vi "VirtualTestInstrument.vi"(8 "error in (no error)":errorcluster, 10 "Message":T1, 11 "RemoteControl":refnum<class "RemoteControl.lvclass">) -> (0 "error out":errorcluster, 2 "processed Message":T1, 3 "RemoteControl":refnum<class "RemoteControl.lvclass">)   [LabVIEW 2016, in "RemoteControl.lvclass"]
uses:
  RemoteControl.lvclass
  Typedefs/Message--Cluster.ctl
  RemoteControl.lvclass/RemoteControl.ctl
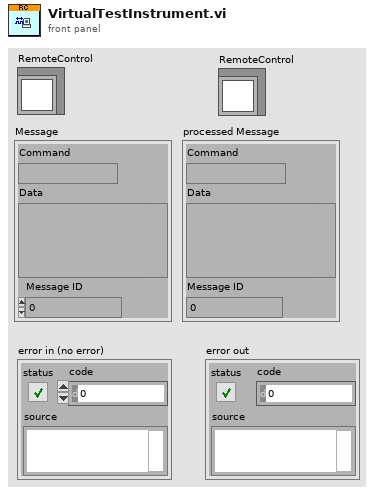
[diagram p1: front panel]
types:
  T1 = typedef "RemoteControl.lvclass/Message--Cluster.ctl" = cluster{"Command":string, "Data":variant, "Message ID":i32}
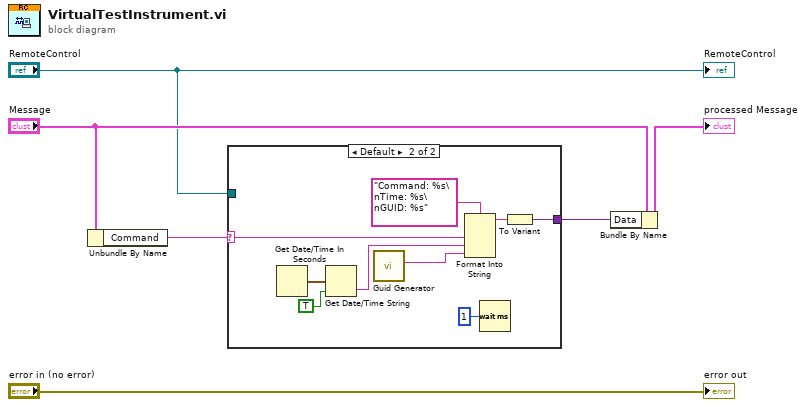
[diagram p0: block diagram]
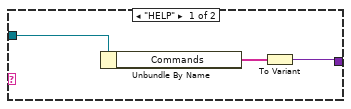
[diagram p2: hidden frame]
diagram:
  n1 = Unbundle By Name("Message") -> ("Command"=w2:string)
  n2 = case shown="Default" w2 {
    selector: w2 -> [_ w11]
    tunnel: [w8 w14] -> w3
    tunnel: "RemoteControl" -> [w7 _]
    frame "HELP" {
      n3 = Unbundle By Name(w7) -> ("Commands"=w9:string[])
      n4 = To Variant(anything=w9) -> (Variant=w8:variant)
    }
    frame Default {
      n5 = Get Date/Time In Seconds() -> (seconds since 1Jan1904=w17:timestamp)
      n6 = Get Date/Time String(seconds (now)=w17, want seconds? (F)=TRUE) -> (time string=w12:string)  [unwired: 1 in, 1 out]
      n7 = call <vilib>:"Guid Generator.vi"() -> ("GUID"=w13:string)  [unwired: 10 in, 1 out]
      n8 = Format Into String(format string="Command: %s\nTime: %s\nGUID: %s", w11, w12, w13) -> (resulting string=w15:string)  [unwired: 2 in, 1 out]
      n9 = Wait (ms)(milliseconds to wait=u32 1) -> ()  [unwired: 1 out]
      n10 = To Variant(anything=w15) -> (Variant=w14:variant)
    }
  }
  n11 = Bundle By Name(cluster="Message", "Data"=w3) -> (→"processed Message":T1)
  "error out" <- "error in (no error)"
  "RemoteControl" <- "RemoteControl"
